vi "Swerve Teleop.vi"(0 "X":dbl, 1 "Rot. Point X":dbl, 3 "Rot. Point Y":dbl, 5 "Y":dbl, 7 "Z":dbl, 11 "Error In":errorcluster, 12 "Robot Centric?":bool=TRUE, 13 "Autonomous?":bool, 14 "Yaw":dbl) -> (4 "Front Left Output":dbl, 6 "Front Right Output":dbl, 8 "Back Left Output":dbl, 10 "Back Right Output":dbl, 15 "Error Out":errorcluster)   [LabVIEW 2016]
uses:
  <vilib>/Rock Robotics/Network Tables/NT Read Number.vi
  <vilib>/Rock Robotics/Network Tables/NT Write Numeric Array.vi
panel:
  in  "Robot Length":dbl=32.0
  in  "Robot Width":dbl=30.0
  # "Swerve Drive Teleoperated Control\nFRC Team 34"
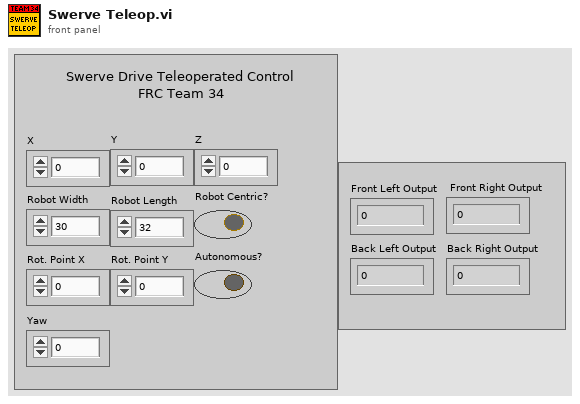
[diagram p1: front panel]
types:
  T1 = enum16{"Front Left", "Front Right", "Back Left", "Back Right"}
  T2 = typedef "WPI_MotorControlDeviceRef.ctl" = cluster{"DeviceStatus":errorcluster, "Type":T3, "PWM":cluster{"PWM Channel":T4, "DeadBand":T5}, "CAN":cluster{"Device Number":u8, "SetOutput VI Ref":variant, "GetOutput VI Ref":variant, "Enable VI Ref":variant, "Disable VI Ref":variant, "Data":variant}, "Invert":bool}
  T3 = typedef "WPI_MotorControlType.ctl" = enum16{"PWM", "CAN"}
  T4 = typedef "FPGA_DIOPWMChannel.ctl" = enum8{"PWM 0", "PWM 1", "PWM 2", "PWM 3", "PWM 4", "PWM 5", "PWM 6", "PWM 7", "PWM 8", "PWM 9", "PWM MXP 0", "PWM MXP 1", "PWM MXP 2", "PWM MXP 3", "PWM MXP 4", "PWM MXP 5", "PWM MXP 6", "PWM MXP 7", "PWM MXP 8", "PWM MXP 9", "Invalid"}
  T5 = typedef "WPI_PWMDeadband.ctl" = cluster{"Name":string, "maxPositivePwm":i32, "minPositivePwm":i32, "centerPwm":i32, "maxNegativePwm":i32, "minNegativePwm":i32, "angularRange":u16}
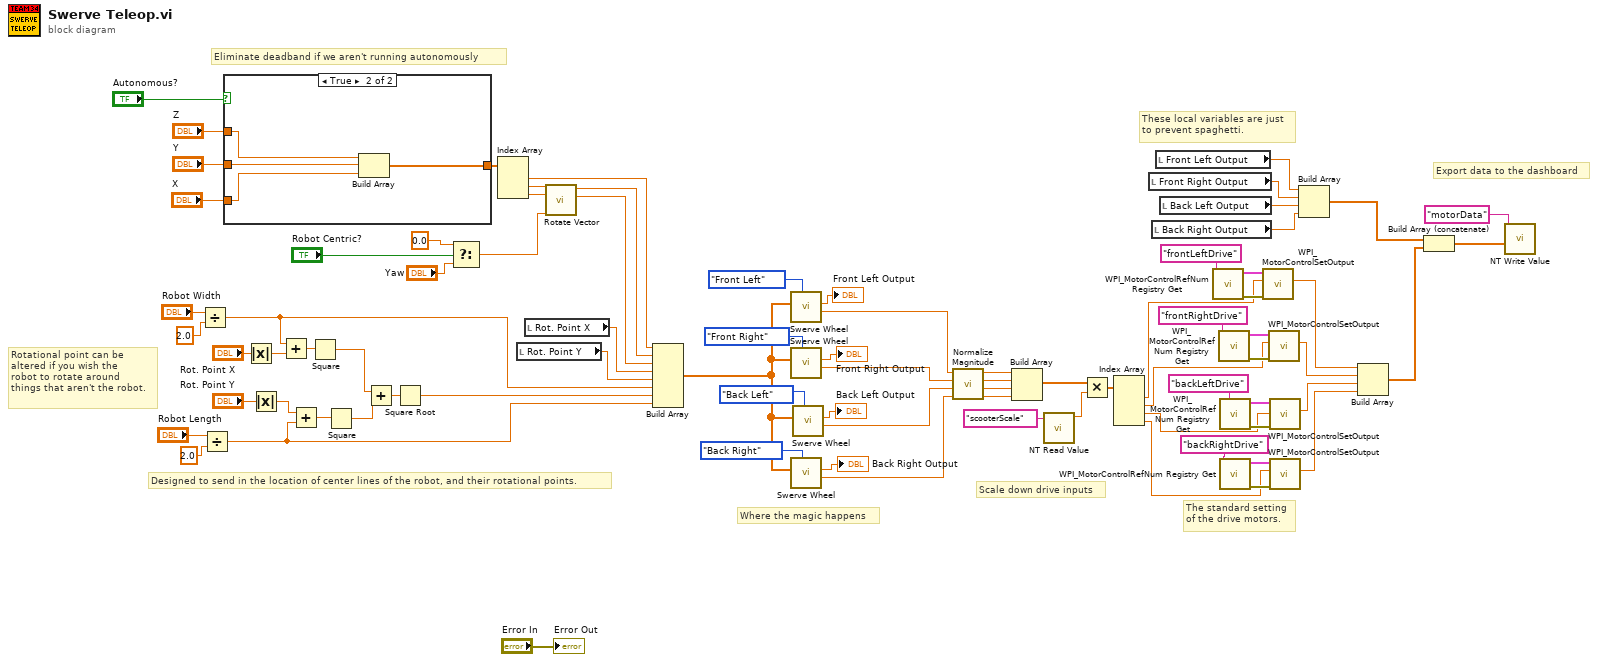
[diagram p0: block diagram]
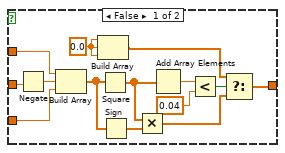
[diagram p2: hidden frame]
diagram:
  # "Rotational point can be \naltered if you wish the \nrobot to rotate around \nthings that aren't the robot."
  # "Scale down drive inputs"
  # "Eliminate deadband if we aren't running autonomously"
  # "These local variables are just \nto prevent spaghetti."
  # "Export data to the dashboard"
  # "Where the magic happens"
  # "The standard setting\nof the drive motors."
  # "Designed to send in the location of center lines of the robot, and their rotational points."
  n1 = Divide(x="Robot Width", y=2.0) -> (x/y=w55:dbl)
  n2 = Divide(x="Robot Length", y=2.0) -> (x/y=w53:dbl)
  n3 = case shown="True" "Autonomous?" {
    tunnel: "Y" -> [w86 w99]
    tunnel: [w85 w97] -> w81
    tunnel: "Z" -> [w84 w100]
    tunnel: "X" -> [w83 w98]
    frame False {
      w92 = 0.0 ("element")
      n4 = Negate(x=w86) -> (-x=w88:dbl)
      n5 = Build Array(w84, w88, w83) -> (w91:dbl[])
      n6 = Build Array(w92, w92, w92) -> (w93:dbl[])
      n7 = Square(x=w91) -> (x^2=w89:dbl[])
      n8 = Sign(1:w91) -> (0:w90:dbl[])
      n9 = Multiply(x=w89, y=w90) -> (x*y=w87:dbl[])
      n10 = Add Array Elements(numeric array=w89) -> (sum=w96:dbl)
      n11 = Less?(x=w96, y=0.04 ("x")) -> (x < y?=w94:bool)
      n12 = Select(t=w93, s=w94, f=w87) -> (s? t:f=w85:dbl[])
    }
    frame True {
      n13 = Build Array(w100, w99, w98) -> (w97:dbl[])
    }
  }
  n14 = Absolute Value(x="Rot. Point X") -> (abs(x)=w67:dbl)
  n15 = Absolute Value(x="Rot. Point Y") -> (abs(x)=w64:dbl)
  n16 = Add(x=w55, y=w67) -> (x+y=w66:dbl)
  n17 = Add(x=w64, y=w53) -> (x+y=w65:dbl)
  n18 = Square(x=w66) -> (x^2=w62:dbl)
  n19 = Square(x=w65) -> (x^2=w63:dbl)
  n20 = Add(x=w62, y=w63) -> (x+y=w61:dbl)
  n21 = Square Root(x=w61) -> (sqrt(x)=w54:dbl)
  n22 = Select(t=0.0, s="Robot Centric?", f="Yaw") -> (s? t:f=w74:dbl)
  n23 = Index Array(array=w81) -> (element #1=w60:dbl, element #2=w76:dbl, element #3=w75:dbl)  [unwired: 3 in]
  n24 = local read "Rot. Point Y"() -> (w56:dbl)
  n25 = local read "Rot. Point X"() -> (w57:dbl)
  n26 = call "Rotate Vector.vi"("Angle"=w74, "X"=w75, "Y"=w76) -> ("X'"=w58:dbl, "Y'"=w59:dbl)  [unwired: 7 in]
  n27 = Build Array(w60, w59, w58, w57, w56, w55, w54, w53) -> (w52:dbl[])
  n28 = call "Swerve Wheel.vi"("Wheel"=T1."Front Left", "Inputs"=w52) -> ("Speed"=w47:dbl, "Motor Output"=→"Front Left Output":dbl)  [unwired: 8 in]
  n29 = call "Swerve Wheel.vi"("Wheel"=T1."Front Right", "Inputs"=w52) -> ("Speed"=w46:dbl, "Motor Output"=→"Front Right Output":dbl)  [unwired: 8 in]
  n30 = call "Swerve Wheel.vi"("Wheel"=T1."Back Right", "Inputs"=w52) -> ("Speed"=w44:dbl, "Motor Output"=→"Back Right Output":dbl)  [unwired: 8 in]
  n31 = call "Swerve Wheel.vi"("Wheel"=T1."Back Left", "Inputs"=w52) -> ("Speed"=w45:dbl, "Motor Output"=→"Back Left Output":dbl)  [unwired: 8 in]
  n32 = call "Normalize Magnitude.vi"("D"=w44, "C"=w45, "B"=w46, "A"=w47) -> ("D'"=w20:dbl, "C'"=w21:dbl, "B'"=w22:dbl, "A'"=w23:dbl)  [unwired: 4 in]
  n33 = Build Array(w23, w22, w21, w20) -> (w19:dbl[])
  n34 = call-poly <vilib>:"NT Read Value.vi"("Name"="scooterScale") -> ("Numeric"=w17:dbl)  [unwired: 9 in, 1 out]
  n35 = Multiply(x=w19, y=w17) -> (x*y=w16:dbl[])
  n36 = Index Array(array=w16) -> (element #1=w15:dbl, element #2=w14:dbl, element #3=w13:dbl, element #4=w12:dbl)  [unwired: 4 in]
  n37 = local read "Front Right Output"() -> (w5:dbl)
  n38 = local read "Back Right Output"() -> (w3:dbl)
  n39 = local read "Front Left Output"() -> (w6:dbl)
  n40 = local read "Back Left Output"() -> (w4:dbl)
  n41 = call <vilib>:"WPI_MotorControlRefNum Registry Get.vi"("refnum name"="frontLeftDrive") -> ("error out"=w42:errorcluster, "MotorControlDevRef"=w41:T2)  [unwired: 9 in]
  n42 = call <vilib>:"WPI_MotorControlRefNum Registry Get.vi"("refnum name"="frontRightDrive") -> ("error out"=w37:errorcluster, "MotorControlDevRef"=w40:T2)  [unwired: 9 in]
  n43 = call <vilib>:"WPI_MotorControlRefNum Registry Get.vi"("refnum name"="backLeftDrive") -> ("error out"=w36:errorcluster, "MotorControlDevRef"=w38:T2)  [unwired: 9 in]
  n44 = call <vilib>:"WPI_MotorControlRefNum Registry Get.vi"("refnum name"="backRightDrive") -> ("error out"=w34:errorcluster, "MotorControlDevRef"=w33:T2)  [unwired: 9 in]
  n45 = call <vilib>:"WPI_MotorControlSetOutput.vi"("error in (no error)"=w42, "Output"=w15, "MotorControlDevRef"=w41) -> ("Motor Output"=w31:dbl)  [unwired: 6 in, 2 out]
  n46 = call <vilib>:"WPI_MotorControlSetOutput.vi"("error in (no error)"=w37, "Output"=w14, "MotorControlDevRef"=w40) -> ("Motor Output"=w30:dbl)  [unwired: 6 in, 2 out]
  n47 = call <vilib>:"WPI_MotorControlSetOutput.vi"("error in (no error)"=w36, "Output"=w13, "MotorControlDevRef"=w38) -> ("Motor Output"=w29:dbl)  [unwired: 6 in, 2 out]
  n48 = call <vilib>:"WPI_MotorControlSetOutput.vi"("error in (no error)"=w34, "Output"=w12, "MotorControlDevRef"=w33) -> ("Motor Output"=w28:dbl)  [unwired: 6 in, 2 out]
  n49 = Build Array(w6, w5, w4, w3) -> (w26:dbl[])
  n50 = Build Array(w31, w30, w29, w28) -> (w27:dbl[])
  n51 = Build Array (concatenate)(w26, w27) -> (w25:dbl[])
  n52 = call-poly <vilib>:"NT Write Value.vi"("Numeric Array"=w25, "Name"="motorData") -> ()  [unwired: 9 in, 1 out]
  "Error Out" <- "Error In"
